vi "Current Write Single.vi"(8 "error in":errorcluster, 9 "Channel Index":i32=1, 10 "Current AV":dbl, 11 "Cycler in":refnum<class "Cycler.lvclass">) -> (0 "error out":errorcluster, 3 "Cycler out":refnum<class "Cycler.lvclass">)   [LabVIEW 2023, in "Cycler.lvclass"]
uses:
  Cycler.lvclass
  Low Level Capabilities/Current/Current Actual Value/Current Actual Value.lvclass
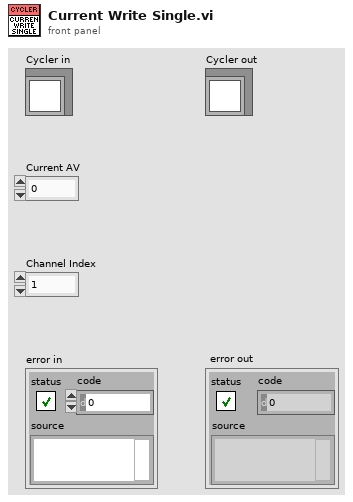
[diagram p1: front panel]
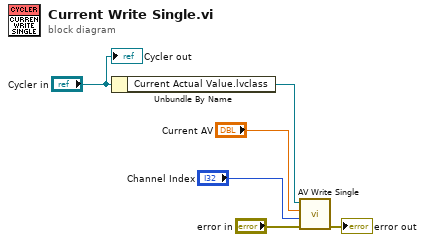
[diagram p0: block diagram]
diagram:
  n1 = Unbundle By Name("Cycler in") -> ("Current Actual Value.lvclass"=w6:refnum<class "Current Actual Value.lvclass">)
  n2 = call-dynamic "AV Write Single.vi"("error in"="error in", "Channel Index"="Channel Index", "Current AV"="Current AV", "Current Actual Value in"=w6) -> ("error out"=→"error out":errorcluster)  [unwired: 6 in, 1 out]
  "Cycler out" <- "Cycler in"
